vi "Actor Core.vi"(8 "error in":errorcluster, 11 "ATM-Controller in":refnum<class "ATM-Controller.lvclass">) -> (0 "error out":errorcluster, 3 "Actor out":refnum<class "Actor.lvclass">)   [LabVIEW 2025, in "ATM-Controller.lvlib" / "ATM-Controller.lvclass"]
doc: "<p>(<strong>Filename</strong>: <span class=\"dnl\">Actor Framework.lvlib:Actor.lvclass:Actor Core.vi</span>)</p>\n<p>Receives messages to the actor, reacts to them, and initiates any error handling that may shut the actor down.</p>\n<p>Descendant classes may override this VI to append parallel tasks for the actor to complete while it handles messages. Overrides use the <a href=\"nihelplauncher://docs/csh?context=lvcore_glang_udclass\">Call Parent Class Method</a> node.</p>"
uses:
  ATM-Controller.lvclass
  C:/Program Files (x86)/National Instruments/LabVIEW 2025/vi.lib/ActorFramework/Actor/Actor.lvclass
  <vilib>/ActorFramework/Actor/Actor.lvclass
  DisplayConsole/DisplayConsole.lvclass
  UserConsole/UserConsole.lvclass
  <vilib>/ActorFramework/Actor/Actor.lvclass/Actor.ctl
  <vilib>/ActorFramework/Message Enqueuer/Message Enqueuer.lvclass/Message Enqueuer.ctl
  ATM-Controller.lvclass/ATM-Controller.ctl
  <vilib>/ActorFramework/Message Enqueuer/Init from Existing Queue.vi
  <vilib>/ActorFramework/Message Enqueuer/Enqueue.vi
  <vilib>/ActorFramework/Stop Msg/Stop Msg.lvclass
  C:/Program Files (x86)/National Instruments/LabVIEW 2025/vi.lib/ActorFramework/Message/Message.lvclass
  <vilib>/ActorFramework/Message Priority Queue/Priority Enqueue.vi
  <vilib>/ActorFramework/Message Enqueuer/Message Enqueuer.lvclass
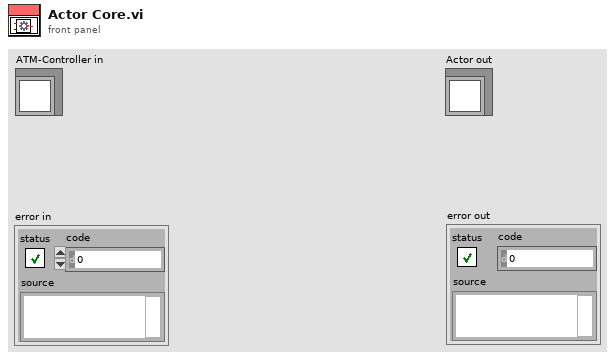
[diagram p1: front panel]
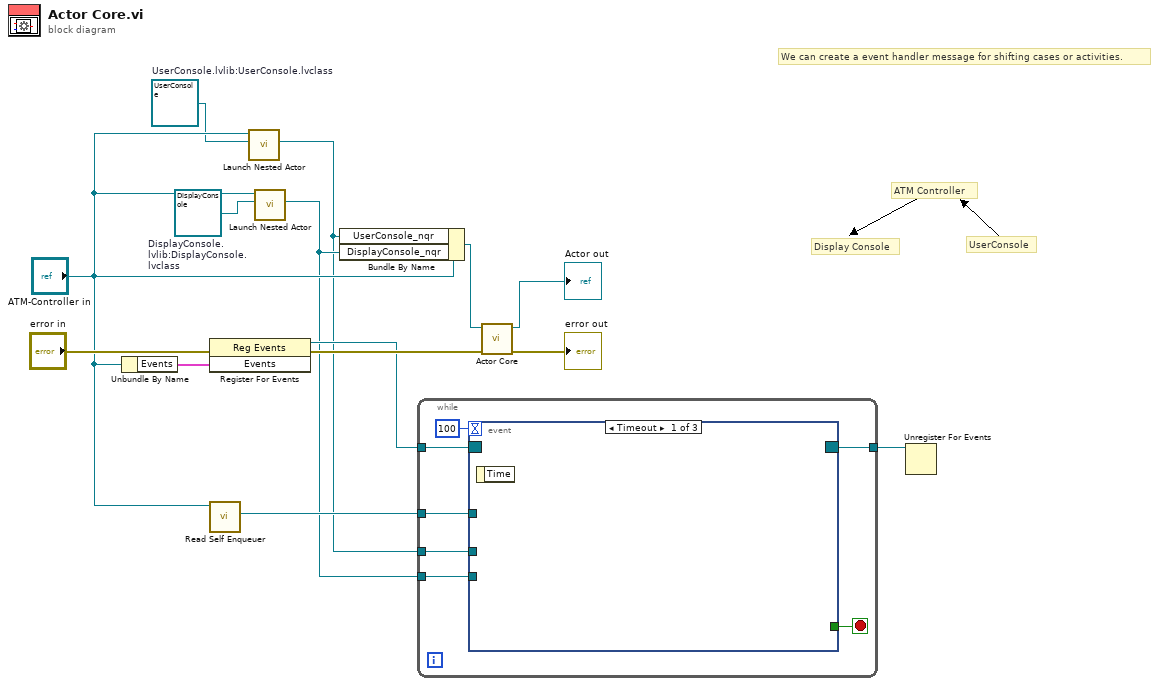
[diagram p0: block diagram]
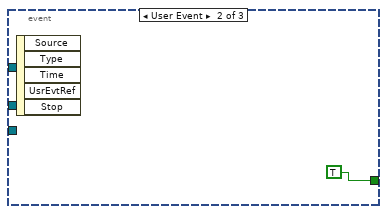
[diagram p2: hidden frame]
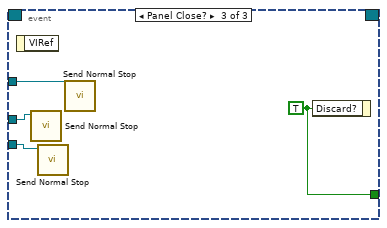
[diagram p3: hidden frame]
diagram:
  w5 = refnum<class "UserConsole.lvclass"> refnum  # UserConsole.lvlib:UserConsole.lvclass
  w4 = refnum<class "DisplayConsole.lvclass"> refnum  # DisplayConsole.lvlib:DisplayConsole.lvclass
  # "Display Console"
  # "UserConsole"
  # "ATM Controller"
  # "We can create a event handler message for shifting cases or activities."
  n1 = Unbundle By Name("ATM-Controller in") -> ("Events"=w9:cluster{"Stop":refnum<user-event>})
  n2 = register-events(error in="error in", w9) -> (reference out=w10:refnum<event-registration>, error out=w11:errorcluster)  [unwired: 1 in]
  n3 = call <vilib>:"Read Self Enqueuer.vi"("Actor"="ATM-Controller in") -> ("Self Enqueuer"=w7:refnum<class "Message Enqueuer.lvclass">)  [unwired: 10 in]
  n4 = call <vilib>:"Launch Nested Actor.vi"("Nested Actor"=w5, "Caller Actor in"="ATM-Controller in") -> ("Nested Actor's Enqueuer"=w1:refnum<class "Message Enqueuer.lvclass">)  [unwired: 7 in, 2 out]
  n5 = call <vilib>:"Launch Nested Actor.vi"("Nested Actor"=w4, "Caller Actor in"="ATM-Controller in") -> ("Nested Actor's Enqueuer"=w2:refnum<class "Message Enqueuer.lvclass">)  [unwired: 7 in, 2 out]
  n6 = Bundle By Name(cluster="ATM-Controller in", "UserConsole_nqr"=w1, "DisplayConsole_nqr"=w2) -> (w3:refnum<class "ATM-Controller.lvclass">)
  n7 = while {
    tunnel: w10 -> [w21]
    tunnel: [w20] -> w8
    tunnel: w7 -> [w18]
    tunnel: w2 -> [w16]
    tunnel: w1 -> [w15]
    stop <- w19 stop-if-true
    n8 = event shown="[0] Timeout" {
      selector: w21 -> [_ _ _]
      dyn-events: [_ _ _] -> w20
      timeout: 100 -> [_ _ _]
      tunnel: [_ TRUE w25] -> w19
      tunnel: w18 -> [_ _ w26]
      tunnel: w16 -> [_ _ w23]
      tunnel: w15 -> [_ _ w24]
      event Timeout {
        n9 = event-data() -> ()  [unwired: 1 in, 1 out]
      }
      event User Event {
        n10 = event-data() -> ()  [unwired: 1 in, 5 out]
      }
      event Panel Close? {
        w25 = TRUE ("Discard?")
        n11 = event-data() -> ()  [unwired: 1 in, 1 out]
        n12 = call <vilib>:"Send Normal Stop.vi"("Message Enqueuer"=w24) -> ()  [unwired: 10 in, 1 out]
        n13 = call <vilib>:"Send Normal Stop.vi"("Message Enqueuer"=w23) -> ()  [unwired: 10 in, 1 out]
        n14 = call <vilib>:"Send Normal Stop.vi"("Message Enqueuer"=w26) -> ()  [unwired: 10 in, 1 out]
        n15 = event-data("Discard?"=w25) -> ()  [unwired: 1 in, 1 out]
      }
    }
  }
  n16 = call-parent "Actor Core.vi"("error in"=w11, "Actor in"=w3) -> ("error out"=→"error out":errorcluster, "Actor out"=→"Actor out":refnum<class "Actor.lvclass">)  [unwired: 8 in]
  n17 = Unregister For Events(event registration refnum=w8) -> ()  [unwired: 1 in, 1 out]
